vi "Tacho Amplitude Measurement.vi"(6 "error in":errorcluster, 7 "samples per channel":i32=1000, 8 "source":tag, 9 "rate":dbl=1000.0 format="%0.2f", 10 "sample mode":i32(ring)=10178 items=["Finite Samples"=10178, "Continuous Samples"=10123, "Hardware Timed Single Point"=12522], 11 "physical channels":tag) -> (0 "error out":errorcluster, 3 "Amplitude Chart":dbl[](graph))   [LabVIEW 2019, in "Part of Main VIs.lvlib" / "Tachometer Library.lvlib"]
uses:
  <vilib>/DAQmx/read.llb/DAQmx Read (Analog 1D DBL 1Chan NSamp).vi
  <vilib>/DAQmx/create/channels.llb/DAQmx Create Channel (AI-Voltage-Basic).vi
  <vilib>/DAQmx/configure/timing.llb/DAQmx Timing (Sample Clock).vi
  <vilib>/DAQmx/miscellaneous.llb/DAQmx Fill In Error Info.vi
  Tachometer Library.lvlib
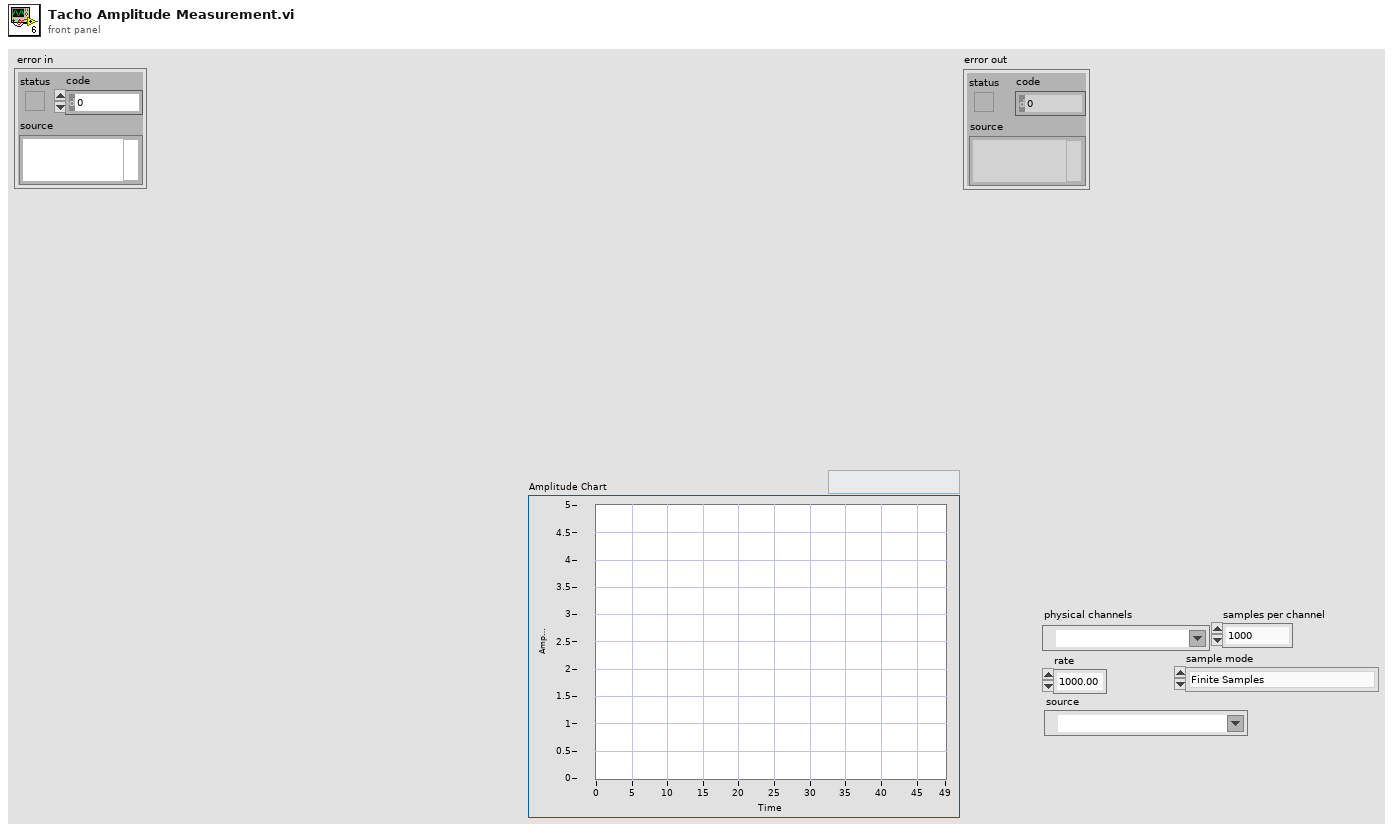
[diagram p1: front panel]
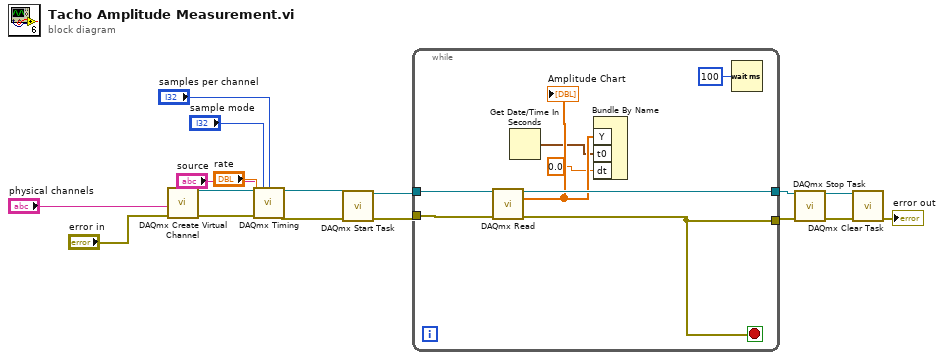
[diagram p0: block diagram]
diagram:
  n1 = call-poly <vilib>:"DAQmx Create Virtual Channel.vi"("physical channels"="physical channels", "error in"="error in") -> ("task out"=w14:refnum<k21>, "error out"=w15:errorcluster)  [unwired: 12 in]
  n2 = call-poly <vilib>:"DAQmx Timing.vi"("task/channels in"=w14, "sample mode"="sample mode", "samples per channel"="samples per channel", "rate"="rate", "source"="source", "error in"=w15) -> ("task out"=w9:refnum<k21>, "error out"=w8:errorcluster)  [unwired: 8 in]
  n3 = call <vilib>:"DAQmx Start Task.vi"("task/channels in"=w9, "error in"=w8) -> ("task out"=w11:refnum<k21>, "error out"=w10:errorcluster)  [unwired: 12 in]
  n4 = while {
    tunnel: w10 -> [w23]
    tunnel: [w18] -> w12
    tunnel: w11 -> [w24]
    tunnel: [w25] -> w13
    stop <- w18 stop-if-true
    n5 = call-poly <vilib>:"DAQmx Read.vi"("task/channels in"=w24, "error in"=w23) -> ("task out"=w25:refnum<k21>, "data"=w21:dbl[], "error out"=w18:errorcluster)  [unwired: 11 in]
    "Amplitude Chart" <- w21
    n6 = Get Date/Time In Seconds() -> (seconds since 1Jan1904=w20:timestamp)
    n7 = Bundle By Name("Y"=w21, "t0"=w20, "dt"=0.0) -> ()  [unwired: 1 in, 1 out]
    n8 = Wait (ms)(milliseconds to wait=u32 100) -> ()  [unwired: 1 out]
  }
  n9 = call <vilib>:"DAQmx Stop Task.vi"("task/channels in"=w13, "error in"=w12) -> ("task out"=w17:refnum<k21>, "error out"=w16:errorcluster)  [unwired: 12 in]
  n10 = call <vilib>:"DAQmx Clear Task.vi"("task in"=w17, "error in"=w16) -> ("error out"=→"error out":errorcluster)  [unwired: 13 in]
